vi "4. Event Based State Machine - Traffic Light Simulator.vi"() -> ()   [LabVIEW 2018]
uses:
  Typedefs/States for Event Based State Machine.ctl
panel:
  in  "stop":bool
  in  "Press Green":bool
  in  "Press Yellow":bool
  in  "Press Red":bool
  out "Yellow":bool
  out "Green":bool
  out "Red":bool
  out "Traffic Lights Picture":picture
  # "Traffic Light Graphic Vector by Vecteezy\n(https://www.vecteezy.com/free-vector/graphic)"
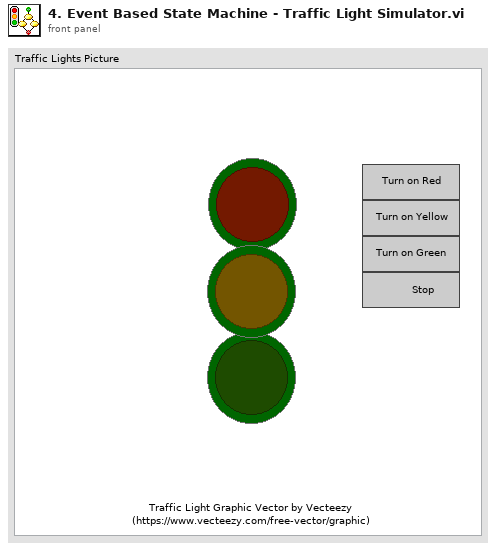
[diagram p1: front panel]
types:
  T1 = cluster{"Wait Before Red":u32, "Wait Before Yellow":u32, "Wait Before Green":u32}
  T2 = typedef "States for Event Based State Machine.ctl" = enum16{"Initialize", "Red", "Yellow", "Green", "Wait for Event", "Stop"}
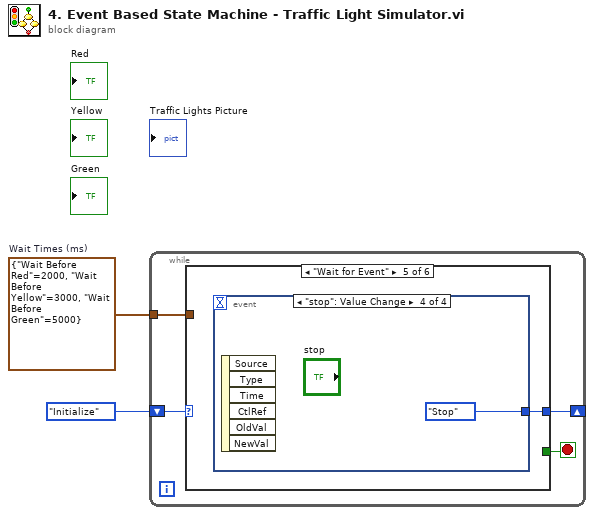
[diagram p0: block diagram]
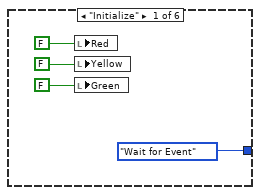
[diagram p2: hidden frame]
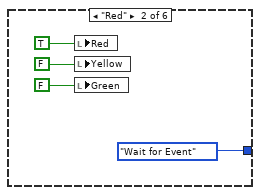
[diagram p3: hidden frame]
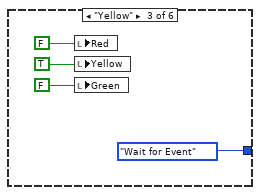
[diagram p4: hidden frame]
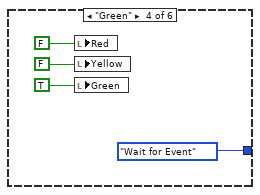
[diagram p5: hidden frame]
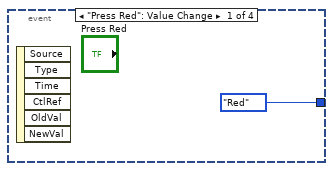
[diagram p6: hidden frame]
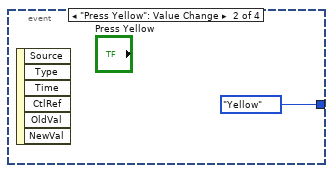
[diagram p7: hidden frame]
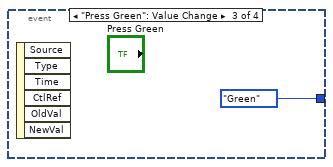
[diagram p8: hidden frame]
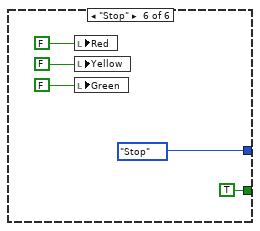
[diagram p9: hidden frame]
diagram:
  w1 = T1 {"Wait Before Red"=2000, "Wait Before Yellow"=3000, "Wait Before Green"=5000}  # Wait Times (ms)
  n1 = while {
    shift-right: [w5] -> _
    shift-left: States_for_Event_Based_State_Machine."Initialize" -> [w6]
    tunnel: w1 -> [w4]
    stop <- w3 stop-if-true
    n2 = case shown="\"Wait for Event\"" w6 {
      tunnel: [States_for_Event_Based_State_Machine."Wait for Event" States_for_Event_Based_State_Machine."Wait for Event" States_for_Event_Based_State_Machine."Wait for Event" States_for_Event_Based_State_Machine."Wait for Event" w23 States_for_Event_Based_State_Machine."Stop"] -> w5
      tunnel: w4 -> [_ _ _ _ _ _]
      tunnel: [_ _ _ _ _ TRUE] -> w3
      frame "Initialize" {
        n3 = local write "Red"(FALSE ("Red")) -> ()
        n4 = local write "Yellow"(FALSE ("Red")) -> ()
        n5 = local write "Green"(FALSE ("Red")) -> ()
      }
      frame "Red" {
        n6 = local write "Red"(TRUE ("Red")) -> ()
        n7 = local write "Yellow"(FALSE ("Red")) -> ()
        n8 = local write "Green"(FALSE ("Red")) -> ()
      }
      frame "Yellow" {
        n9 = local write "Red"(FALSE ("Red")) -> ()
        n10 = local write "Yellow"(TRUE ("Red")) -> ()
        n11 = local write "Green"(FALSE ("Red")) -> ()
      }
      frame "Green" {
        n12 = local write "Red"(FALSE ("Red")) -> ()
        n13 = local write "Yellow"(FALSE ("Red")) -> ()
        n14 = local write "Green"(TRUE ("Red")) -> ()
      }
      frame "Wait for Event" {
        n15 = event shown="[3] \"stop\": Value Change" {
          selector: _ -> [_ _ _ _]
          dyn-events: _ -> [_ _ _ _]
          timeout: _ -> [_ _ _ _]
          tunnel: [States_for_Event_Based_State_Machine."Red" States_for_Event_Based_State_Machine."Yellow" States_for_Event_Based_State_Machine."Green" States_for_Event_Based_State_Machine."Stop"] -> w23
          event "Press Red": Value Change {
            n16 = event-data() -> ()  [unwired: 1 in, 6 out]
          }
          event "Press Yellow": Value Change {
            n17 = event-data() -> ()  [unwired: 1 in, 6 out]
          }
          event "Press Green": Value Change {
            n18 = event-data() -> ()  [unwired: 1 in, 6 out]
          }
          event "stop": Value Change {
            n19 = event-data() -> ()  [unwired: 1 in, 6 out]
          }
        }
      }
      frame "Stop" {
        n20 = local write "Red"(FALSE ("Red")) -> ()
        n21 = local write "Yellow"(FALSE ("Red")) -> ()
        n22 = local write "Green"(FALSE ("Red")) -> ()
      }
    }
  }
